vi "CollectData.vi"(8 "error in (no error)":errorcluster, 11 "Novatech in":refnum<class "Novatech.lvclass">) -> (0 "error out":errorcluster, 3 "Novatech out":refnum<class "Novatech.lvclass">)   [LabVIEW 2013, in "Novatech.lvclass"]
uses:
  Novatech.lvclass
  Device/Device.lvclass
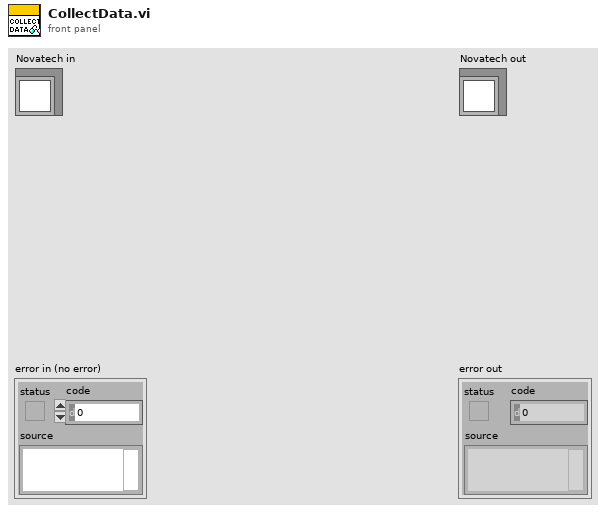
[diagram p1: front panel]
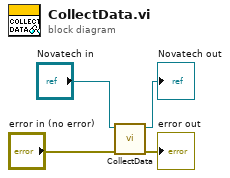
[diagram p0: block diagram]
diagram:
  n1 = call-parent "CollectData.vi"("error in (no error)"="error in (no error)", "Device in"="Novatech in") -> ("error out"=→"error out":errorcluster, "Device out"=→"Novatech out":refnum<class "Novatech.lvclass">)  [unwired: 8 in]
